vi "sub vi - AI test v1.vi"(10 "stop":bool) -> (0 "error out":errorcluster)   [LabVIEW 2013]
uses:
  <vilib>/Platform/TimedLoop/XDataNode/timing_clust.ctl
  <vilib>/Platform/TimedLoop/XDataNode/nitl_modes.ctl
  <vilib>/Platform/TimedLoop/XDataNode/wakeup.ctl
  <vilib>/platform/TimedLoop/XDataNode/XDataNode.xnode
  <vilib>/Platform/TimedLoop/XDataNode/XDNodeRunTimeDep.lvlib
panel:
  out "CH 7":dbl
  in  "SAMPLES":dbl
  in  "RATE":dbl
  out "Waveform Graph":dynamicdata(graph)
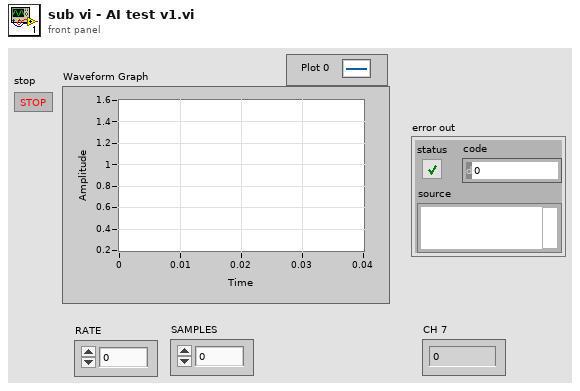
[diagram p1: front panel]
types:
  T1 = typedef "XDNodeRunTimeDep.lvlib/timing_clust.ctl" = cluster{"Expected End [f-1]":u64, "Actual End [f-1]":u64, "Finished Late? [f-1]":bool, "Expected End [i-1]":u64, "Actual End [i-1]":u64, "Finished Late? [i-1]":bool, "Expected Start [i]":u64, "Actual Start [i]":u64, "Expected Start [f]":u64, "Actual Start [f]":u64, "Source Name":string, "Structure Name":string, "Period":i64, "Deadline":i64, "Offset":i64, "Start":i64, "Priority":i32, "Timeout":i32, "Mode":T2, "Wakeup Reason":T3, "Error":errorcluster, "Source Type":string, "Secondary Source Type":string, "Global End Time":u64, "Global Start Time":u64, "Frame Duration":u64, "Iteration Duration":u64, "Assigned CPU":i32, "I/O Scan Engine Mode":u32}
  T2 = typedef "XDNodeRunTimeDep.lvlib/nitl_modes.ctl" = enum32{"No Change", "Process missed periods, maintain original phase", "Discard missed periods, maintain original phase", "Process missed periods, ignore original phase", "Discard missed periods, ignore original phase"}
  T3 = typedef "XDNodeRunTimeDep.lvlib/wakeup.ctl" = enum32{"Normal", "Aborted", "Asynchronous wakeup", "Timing source error", "Timed loop error", "Timeout"}
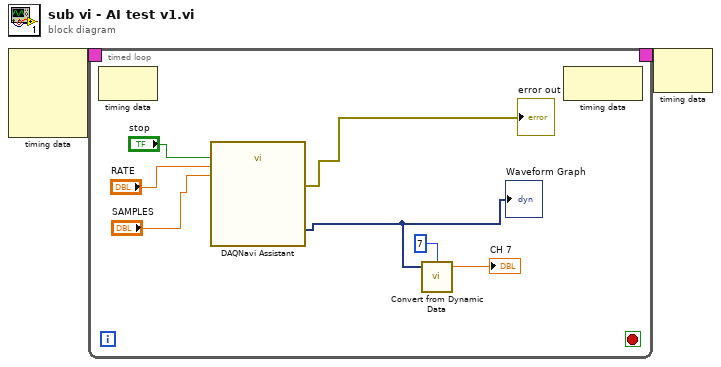
[diagram p0: block diagram]
diagram:
  n1 = node-c288() -> (w2:T1)  [unwired: 4 in]
  n2 = timed-loop {
    timing: w2 -> [_]
    timing-out: [_] -> w1
    stop <- _ stop-if-true
    n3 = node-c288() -> ()  [unwired: 1 in, 1 out]
    n4 = call "DAQNavi Assistant"("stop(true)"="stop", "conversion rate(Hz)"="RATE", "samples"="SAMPLES") -> ("error out"=→"error out":errorcluster, "data out(DDT)"=w5:dynamicdata)  [unwired: 23 in]
    "Waveform Graph" <- w5
    n5 = call "Convert from Dynamic Data"("Dynamic Data Type"=w5, "Channel"=7) -> ("Scalar"=→"CH 7":dbl)  [unwired: 2 in]
    n6 = node-c288() -> ()  [unwired: 1 in, 1 out]
  }
  n7 = node-c288(w1) -> ()  [unwired: 1 out]
